vi "Can_TransferData.vi"(10 "Seq?":bool, 11 "Data":T1 {"payload" format="%02x"; "identifier" format="%x"}) -> (3 "Data":T1 {"payload" format="%02x"; "identifier" format="%x"})   [LabVIEW 2015]
uses:
  Crl/Can_DataType.ctl
panel:
  # "ms"
  # "ms"
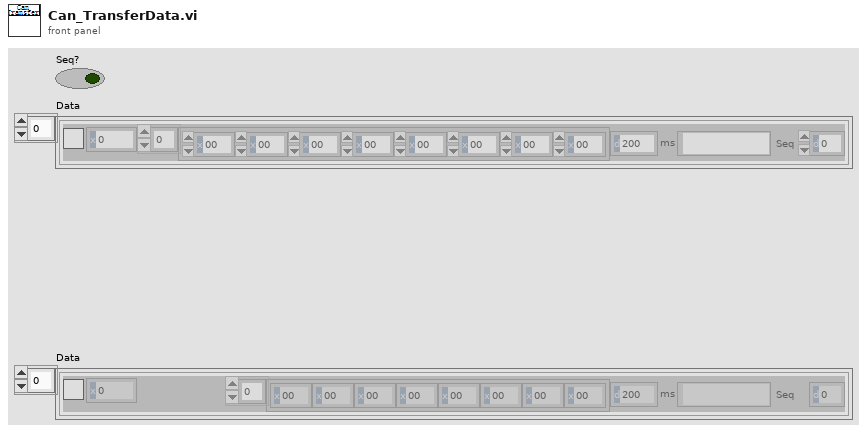
[diagram p1: front panel]
types:
  T1 = typedef "Can_DataType.ctl" = cluster{"identifier":u32, "payload":u8[], "Send?":bool, "Note":string, "Delays":u32, "Seq":i32}[]
  T2 = cluster{"identifier":u32, "payload":u8[], "Send?":bool, "Note":string, "Delays":u32, "Seq":i32}[]
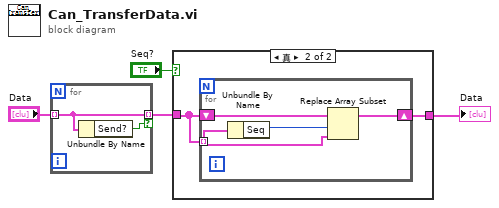
[diagram p0: block diagram]
diagram:
  n1 = for {
    tunnel: [w5] -> w2 mode=indexing if=w6
    tunnel: "Data" -> [w5] mode=indexing
    n2 = Unbundle By Name(w5) -> ("Send?"=w6:bool)
  }
  n3 = case shown="真" "Seq?" {
    tunnel: w2 -> [w7 w9]
    tunnel: [w7 w8] -> w1
    frame False {
    }
    frame True {
      n4 = for {
        tunnel: w9 -> [w11] mode=indexing
        shift-right: [w10] -> w8
        shift-left: w9 -> [w13]
        n5 = Unbundle By Name(w11) -> ("Seq"=w12:i32)
        n6 = Replace Array Subset(array=w13, new element=w11, index=w12) -> (w10:T2)
      }
    }
  }
  "Data" <- w1
